vi "tsfifo_clear_canfd_receive_buffers.vi"(8 "error in (no error)":errorcluster caption="错误输入（无错误）", 10 "AIdxChn":i32, 11 "路径输入":path) -> (0 "error out":errorcluster caption="错误输出", 2 "function return":i32, 3 "路径输出":path)   [LabVIEW 2014]
doc: "Function Introduction :\nClear the cached messages in the CANFD channel\nCall location :\nBefore executing the interaction protocol (such as UDS diagnosis), first call this command to cache the\nClear historical data\ninput parameter :\nAChn: Hardware Channel\nReturn value :\nReturn the number of CAN messages in the cache"
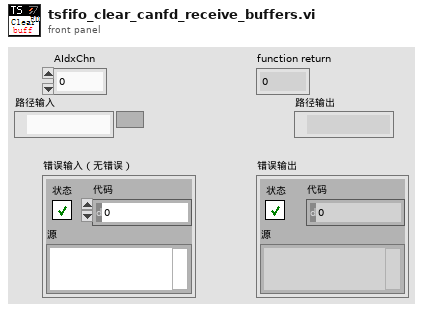
[diagram p1: front panel]
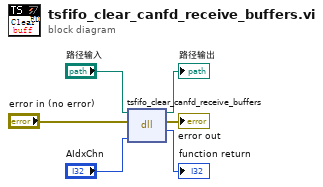
[diagram p0: block diagram]
diagram:
  n1 = dll-call lib="D:/Work/LabVIEW Code/TSMaster Labview SDK/LabVIEW/LabVIEW-TSMasterAPI_CLN/TSMasterAPI_LabVIEW-2024-08-20 14-08-34/Not_organized_vi/TSMaster.*" fn="tsfifo_clear_canfd_receive_buffers"(path in="路径输入", error in="error in (no error)", "AIdxChn"="AIdxChn") -> (path out=→"路径输出":path, error out=→"error out":errorcluster, "返回类型"=→"function return":i32)  [unwired: 2 in]
